vi "DPT Save to Excel.vi"(4 "2015 Raw Data":string[][](array[string]), 6 "Summary":string="*****  2015 DRYER D.O.E. AUDIT DATA WORKSHEET   *****\n\n    Technician:  Corey\t\t\t\tModel #: GSH25J\n    Date:  11/19/1984\t\t\t                Serial #: 96060225101          \t\t\n    Energy Cloth Type:\t  ____________\t\tMfg Date: ____________         \t\n    Blower Type:  _________________\t\tRm. Dry Bulb: F       \n    Blower Dia:  ____________  IN\t\tRm. Wet Bulb:____________F         \n    Airflow (AHAM Sim):  _______CFM\t\tRm. Rel Humidity:   %       \n    Drying Cycle:  ________________\t\tHIGH HEAT_________________________\n    Load Cycles:  \t                (LIMIT 25, WEIGH BONE DRY EVERY 5th RUN)\n    Washer Water Temperature ( 60 ± 5°F ): \n    Exhaust Type: \n    Equipment Calibration: Reference Spreadsheet File\n\n    \tTotal Drying Time:     41.7  min\n(A) \tBone Dry Weight:       8.338 lb\t\t\t(ALL WEIGHTS FROM REF SCALE)\n(B) \tInitial Wt. Wet Load:  13.126  lb\t\t(C) Initial Ret. 100*(B-A)/A:  57.42 %\n(D) \tFinal Wt. Dried Load:  8.686  lb\t\t(E) Final Ret.   100*(D-A)/A:  4.17 %\n\nELECTRICAL ENERGY:\n\n(F) Electrical Energy Used:  0.139  kwh\n\nGAS ENERGY:\n\n\tGas Meter Temp:   73.400 F\t   (H) Gas Corr. Factor:     0.810  ++ \n\tGas Meter Press:  7.700 in H20      (J) Gas Heating Value:    1010.0  BTU/CUFT           \n(G) Metered Gas Vol:      248.500 Liters (K) Gas Energy (G*H*J*0.0353):     7182.0 BTU\t     \n           \nBarometer Press:  24.362 in HG\t           Supply Voltage: \t\n\nReference Pressure: 14.730                    Reference Temperature: 60.0\n\n++ From PC program per US Bureau of Stds, C417,1938\n \n(N) Total Energy (Gas + Electric) (kWh): 2.242\n    [(K/3415)+F]\n\n(L) Per cycle Total Electric Energy Consumption adjusted to 4%:  2.343 KWH/CYCLE\n    ([53.5/(C-E)]*1.04*N)\n\n(I) Per Cycle Off Mode/Standby Mode Power: 0.12\n    [V/(1000*283)*8620] \n\n(V) Standby Mode Power: 3.960 Watts\n    Off Mode Power: 0.000 Watts \n         Off Mode > 0  Standby Mode > 0: [0.5*(Off Mode+Standby Mode)]\n         Off Mode > 0  Standby Mode = 0: [(Off Mode+Standby Mode)]\n\n(E60) Annual Consumption: [(L*283)]  663 kwh\n\n(R) Combined Energy Factor: [A/(L+I)] 3.384\n\n***********************************************************\n   * (P) Per Cycle Energy Efficiency (A/L): 3.559\n***********************************************************", 7 "Pass Fail Lab Eval":string, 8 "error in (no error)":errorcluster, 9 "FileInit Cluster":T1={"Dryer Type"="NR", "TR Number"="", "Lab ID"="", "Output Stream Header"=[], "Stream Data Output"=[], "2015 Array"=[], "Dryer Test Data"=[], "Off Mode Array"=[], "Calibration Array"=[], "File Initialization Array"=[], "Load Run Number"="", "Model:"="DGnn", "Serial Number:"="DGnn", "Build:"="", "Test_Title Per TR:"="HeatUP", "Ambient Temp SetPoint:"="70", "Washer Water \nTemperature ( 60 ± 5°F ):"="60", "Frequency:"="60 HZ", "Dryness Setting:"="", "Heat Setting:"="", "Ambient RH:"="50", "Drying Cycle:"="", "Exhaust:"="NR", "Comments:"="", "Technician:"="", "Engineer:"="CraigT.", "Water Hardness (PPM)"="60", "Empty Dryer Cold Weight"="HeatUP", "Date:"="DGnn", "Version:"="DGnn", "Computer:"="1A", "Load Type"="", "Nominal Load  Weight"="", "Weights Out"={"Measured IMC"=7.0, "Actual RMC"=7.0, "RMC (Desired)"=100.0, "Bone Dry Wt(lbs)"=7.0, "Tolerance(%)"=5.0}, "Test Station:"="1A", "Heat Setting:"="", "Dryness Setting:"="", "Frequency:"="60 HZ", "Water Hardness (PPM)"="60", "Washer Water \nTemperature ( 60 ± 5°F )"="60", "Flow Computer Info Baro,BTUF,u,Z"=[], "Filename"="", "Analog Voltage Data"=[]} {"Weights Out"."Tolerance(%)" format="%0#_6g"; "Weights Out"."Bone Dry Wt(lbs)" format="%03_6g"; "Weights Out"."RMC (Desired)" format="%0#_6g"; "Weights Out"."Actual RMC" format="%03_6g"; "Weights Out"."Measured IMC" format="%0#_6g"}, 10 "report file path":path, 11 "template (empty)":path) -> (0 "error out":errorcluster, 3 "Error":errorcluster[](array[cluster]))   [LabVIEW 2016]
uses:
  Utility/Save File/File Setup (Public)/Type Definition/DPT Output Dryer Information.ctl
  <vilib>/addons/_office/_exclsub.llb/font.ctl
  <vilib>/addons/_office/excel.llb/Excel Easy Table (str).vi
  <vilib>/Utility/NIReport.llb/NI_report.lvclass
  <vilib>/Utility/NIReport.llb/Excel/NI_Excel.lvclass
  <vilib>/addons/_office/NI_ReportGenerationToolkit.lvlib
  Utility/Save File/File Setup.lvlib
panel:
  in  "Machine Debug Information":string[][](array[string])
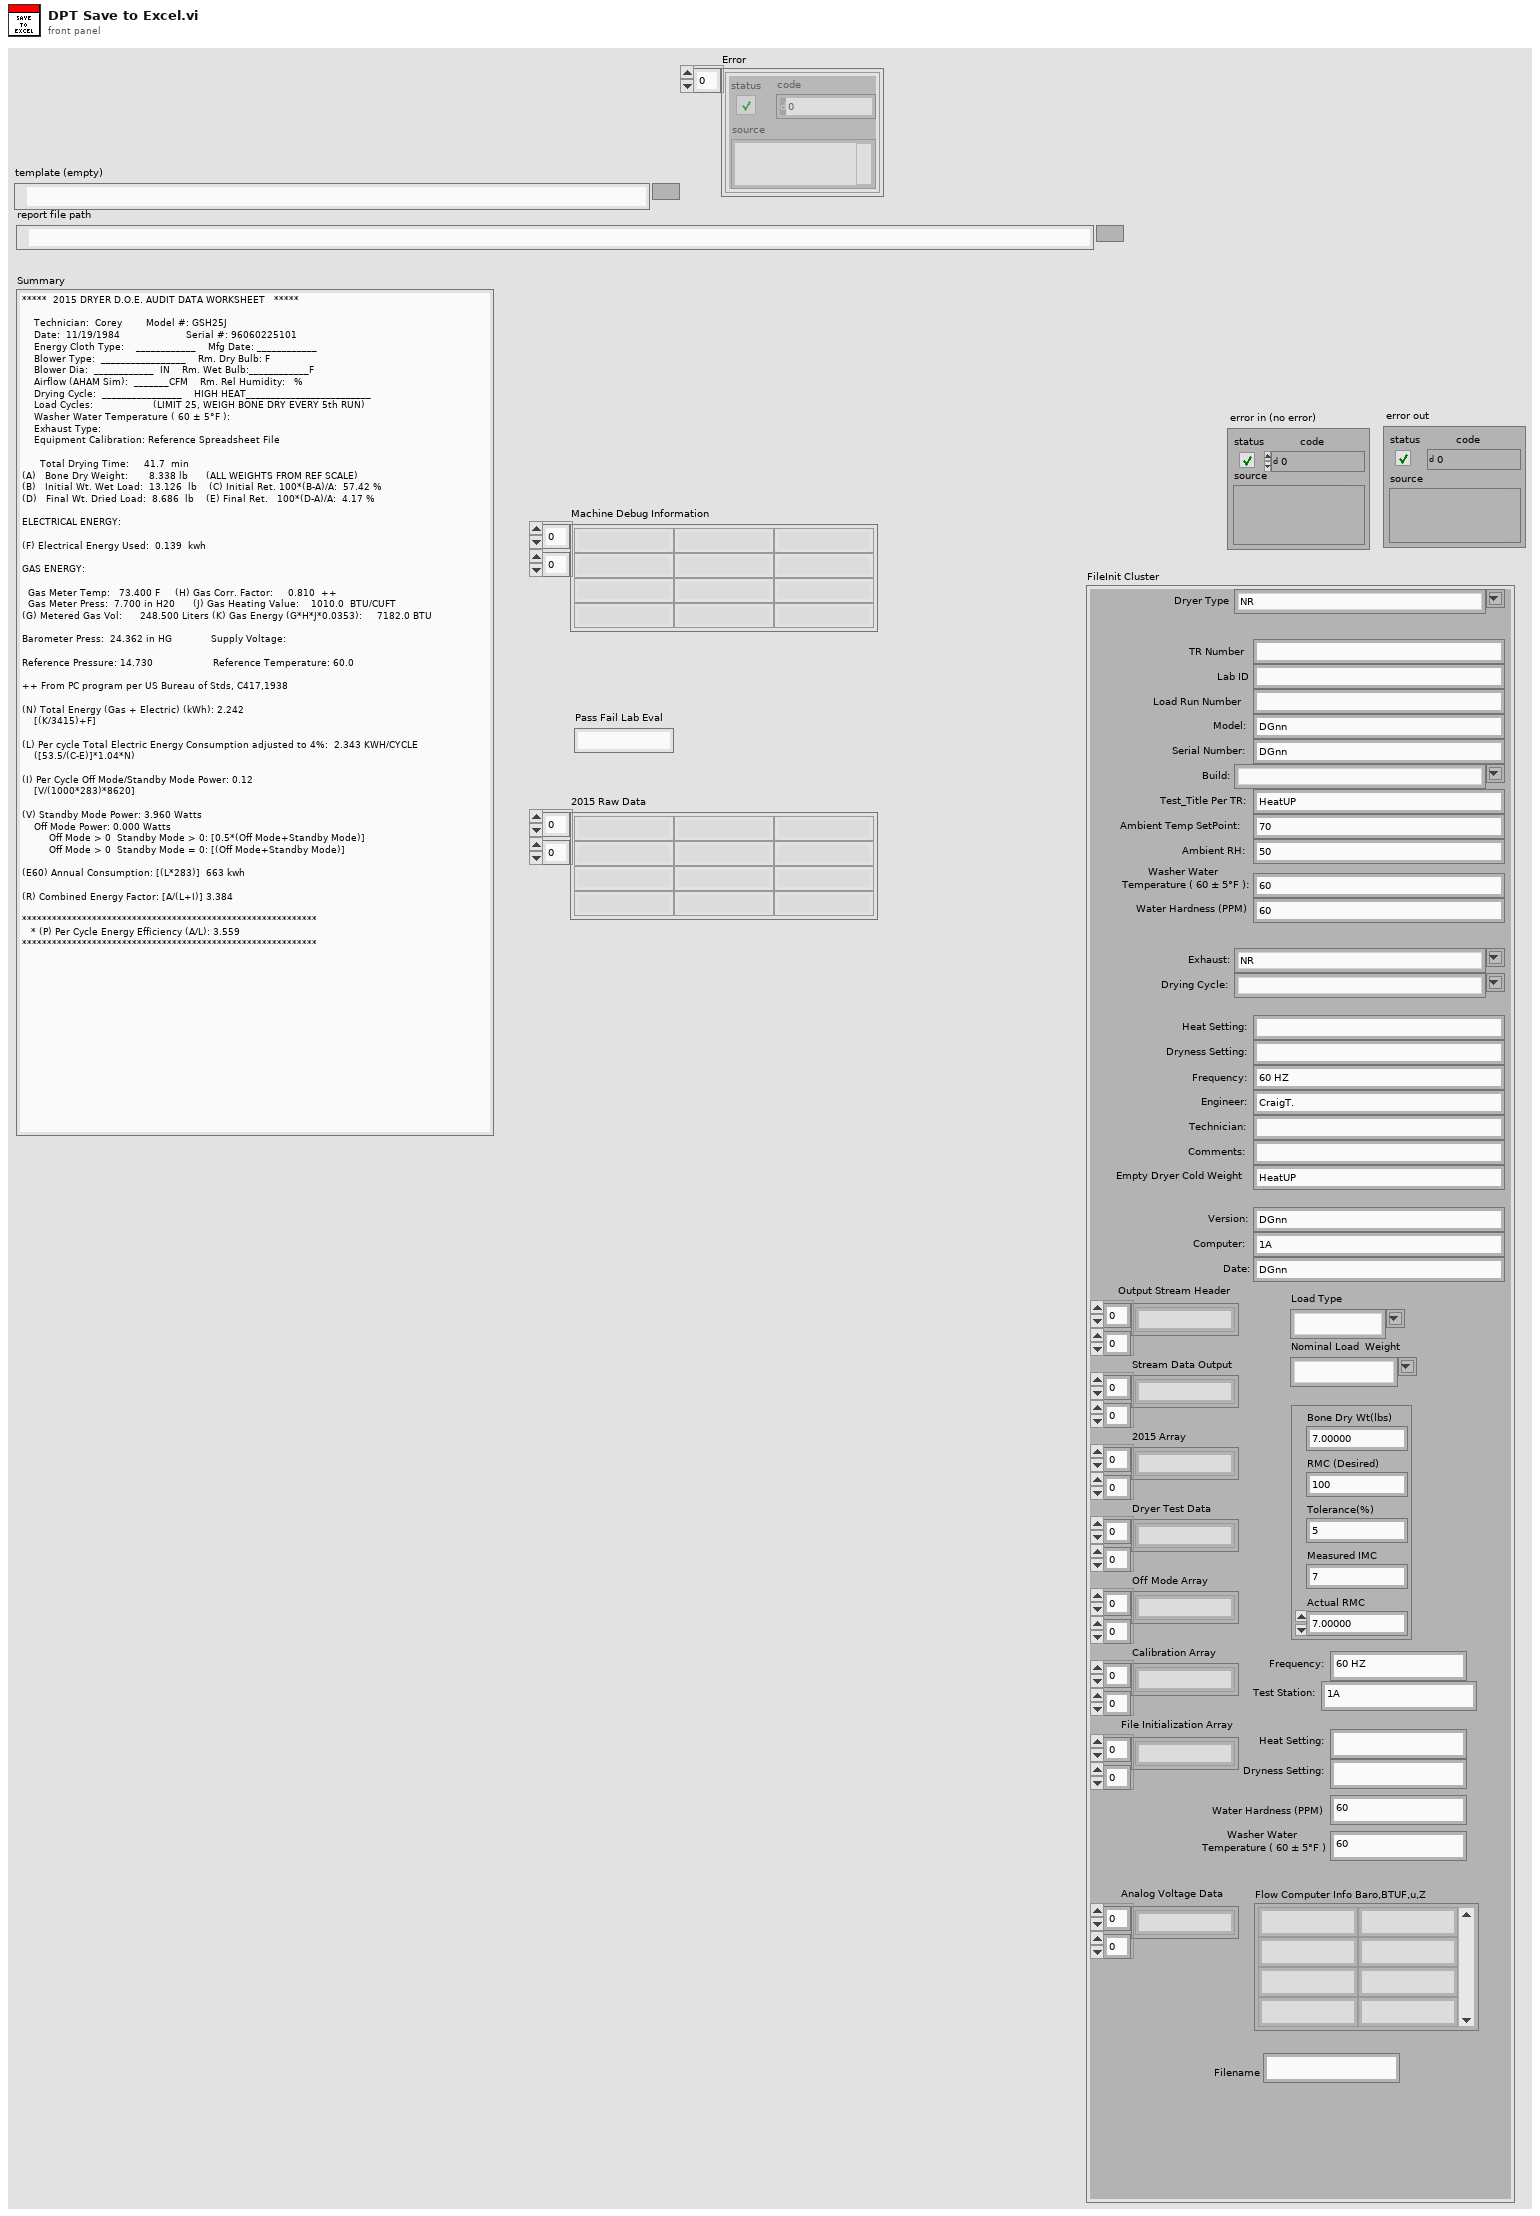
[diagram p1: front panel]
types:
  T1 = typedef "File Setup.lvlib/DPT Output Dryer Information.ctl" = cluster{"Dryer Type":string, "TR Number":string, "Lab ID":string, "Output Stream Header":string[][], "Stream Data Output":string[][], "2015 Array":string[][], "Dryer Test Data":string[][], "Off Mode Array":string[][], "Calibration Array":string[][], "File Initialization Array":string[][], "Load Run Number":string, "Model:":string, "Serial Number:":string, "Build:":string, "Test_Title Per TR:":string, "Ambient Temp SetPoint:":string, "Washer Water \nTemperature ( 60 ± 5°F ):":string, "Frequency:":string, "Dryness Setting:":string, "Heat Setting:":string, "Ambient RH:":string, "Drying Cycle:":string, "Exhaust:":string, "Comments:":string, "Technician:":string, "Engineer:":string, "Water Hardness (PPM)":string, "Empty Dryer Cold Weight":string, "Date:":string, "Version:":string, "Computer:":string, "Load Type":string, "Nominal Load  Weight":string, "Weights Out":cluster{"Measured IMC":dbl, "Actual RMC":dbl, "RMC (Desired)":dbl, "Bone Dry Wt(lbs)":dbl, "Tolerance(%)":dbl}, "Test Station:":string, "Heat Setting:":string, "Dryness Setting:":string, "Frequency:":string, "Water Hardness (PPM)":string, "Washer Water \nTemperature ( 60 ± 5°F )":string, "Flow Computer Info Baro,BTUF,u,Z":string[][], "Filename":string, "Analog Voltage Data":string[][]}
  T2 = typedef "NI_ReportGenerationToolkit.lvlib/font.ctl" = cluster{"font name":string, "font size":dbl, "bold":u16, "italic":u16, "underline":u16, "strike through":u16, "font color":u32}
  T3 = enum16{"maximized", "minimized", "normal", "no change"}
  T4 = enum16{"Standard Report", "HTML", "Word", "Excel"}
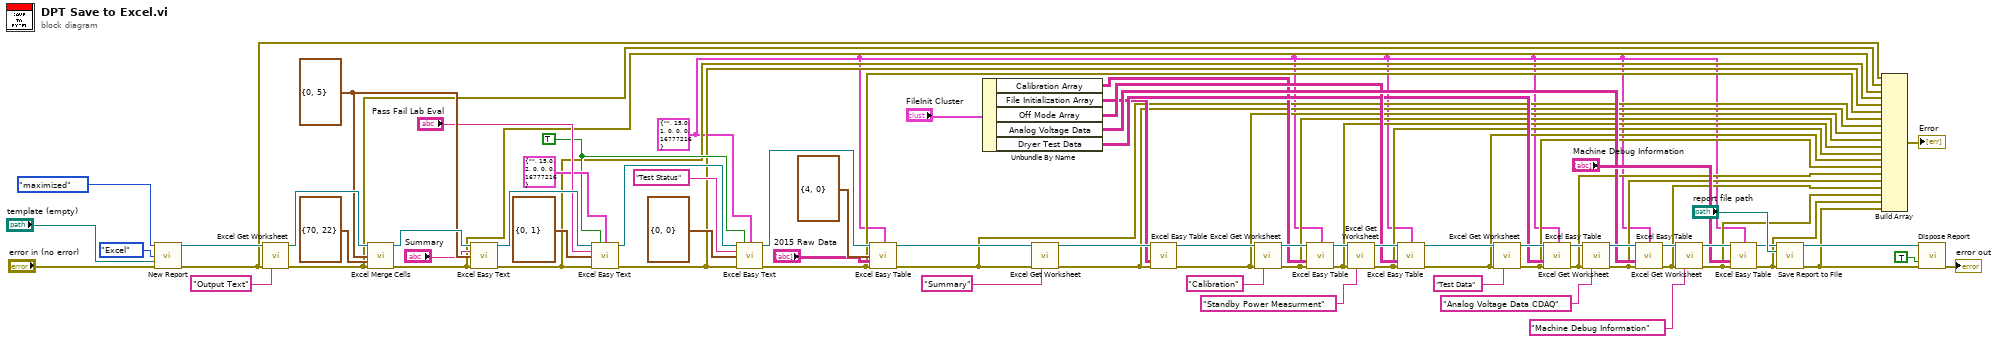
[diagram p0: block diagram]
diagram:
  w1 = T2 {"font name"="", "font size"=15.0, "bold"=1, "italic"=0, "underline"=0, "strike through"=0, "font color"=16777216} ("font")
  w42 = TRUE ("border? (F)")
  w64 = cluster{"row":i32, "column":i32} {"row"=0, "column"=5} ("start (-1, -1)")
  n1 = call <vilib>:"New Report.vi"("window state (normal)"=T3."maximized", "report type"=T4."Excel", "template (empty)"="template (empty)", "error in (no error)"="error in (no error)") -> ("report out"=w68:refnum<class "NI_report.lvclass">, "error out"=w22:errorcluster)  [unwired: 10 in]
  n2 = call <vilib>:"Excel Get Worksheet.vi"("report in"=w68, "error in (no error)"=w22, "name (\"\")"="Output Text" ("name (\"\")")) -> ("report out"=w67:refnum<class "NI_report.lvclass">, "error out"=w21:errorcluster)  [unwired: 11 in]
  n3 = call <vilib>:"Excel Merge Cells.vi"("report in"=w67, "start (-1, -1)"=w64, "end (-1, -1)"=cluster{"row":i32, "column":i32} {"row"=70, "column"=22}, "error in (no error)"=w21) -> ("report out"=w65:refnum<class "NI_report.lvclass">, "error out"=w20:errorcluster)  [unwired: 10 in]
  n4 = call <vilib>:"Excel Easy Text.vi"("report in"=w65, "text"="Summary", "start (-1, -1)"=w64, "error in (no error)"=w20) -> ("report out"=w62:refnum<class "NI_report.lvclass">, "error out"=w19:errorcluster)  [unwired: 7 in, 3 out]
  n5 = call <vilib>:"Excel Easy Text.vi"("report in"=w62, "border? (F)"=w42, "font"=T2 {"font name"="", "font size"=15.0, "bold"=2, "italic"=0, "underline"=0, "strike through"=0, "font color"=16777216}, "text"="Pass Fail Lab Eval", "start (-1, -1)"=cluster{"row":i32, "column":i32} {"row"=0, "column"=1}, "error in (no error)"=w19) -> ("report out"=w43:refnum<class "NI_report.lvclass">, "error out"=w18:errorcluster)  [unwired: 5 in, 3 out]
  n6 = call <vilib>:"Excel Easy Text.vi"("report in"=w43, "border? (F)"=w42, "font"=w1, "text"="Test Status", "start (-1, -1)"=cluster{"row":i32, "column":i32} {"row"=0, "column"=0}, "error in (no error)"=w18) -> ("report out"=w26:refnum<class "NI_report.lvclass">, "error out"=w17:errorcluster)  [unwired: 5 in, 3 out]
  n7 = call-poly <vilib>:"Excel Easy Table.vi"("report in"=w26, "font"=w1, "start (0, 0)"=cluster{"row":i32, "column":i32} {"row"=4, "column"=0}, "text data"="2015 Raw Data", "error in (no error)"=w17) -> ("report out"=w25:refnum<class "NI_report.lvclass">, "error out"=w16:errorcluster)  [unwired: 6 in, 3 out]
  n8 = Unbundle By Name("FileInit Cluster") -> ("Calibration Array"=w30:string[][], "File Initialization Array"=w34:string[][], "Off Mode Array"=w38:string[][], "Analog Voltage Data"=w39:string[][], "Dryer Test Data"=w37:string[][])
  n9 = call <vilib>:"Excel Get Worksheet.vi"("report in"=w25, "error in (no error)"=w16, "name (\"\")"="Summary" ("name (\"\")")) -> ("report out"=w35:refnum<class "NI_report.lvclass">, "error out"=w15:errorcluster)  [unwired: 11 in]
  n10 = call-poly <vilib>:"Excel Easy Table.vi"("report in"=w35, "text data"=w34, "error in (no error)"=w15) -> ("report out"=w33:refnum<class "NI_report.lvclass">, "error out"=w14:errorcluster)  [unwired: 8 in, 3 out]
  n11 = call <vilib>:"Excel Get Worksheet.vi"("report in"=w33, "error in (no error)"=w14, "name (\"\")"="Calibration" ("name (\"\")")) -> ("report out"=w31:refnum<class "NI_report.lvclass">, "error out"=w13:errorcluster)  [unwired: 11 in]
  n12 = call-poly <vilib>:"Excel Easy Table.vi"("report in"=w31, "font"=w1, "text data"=w30, "error in (no error)"=w13) -> ("report out"=w29:refnum<class "NI_report.lvclass">, "error out"=w12:errorcluster)  [unwired: 7 in, 3 out]
  n13 = call <vilib>:"Excel Get Worksheet.vi"("report in"=w29, "error in (no error)"=w12, "name (\"\")"="Standby Power Measurment" ("name (\"\")")) -> ("report out"=w59:refnum<class "NI_report.lvclass">, "error out"=w11:errorcluster)  [unwired: 11 in]
  n14 = call-poly <vilib>:"Excel Easy Table.vi"("report in"=w59, "font"=w1, "text data"=w38, "error in (no error)"=w11) -> ("report out"=w47:refnum<class "NI_report.lvclass">, "error out"=w10:errorcluster)  [unwired: 7 in, 3 out]
  n15 = call <vilib>:"Excel Get Worksheet.vi"("report in"=w47, "error in (no error)"=w10, "name (\"\")"="Test Data" ("name (\"\")")) -> ("report out"=w56:refnum<class "NI_report.lvclass">, "error out"=w9:errorcluster)  [unwired: 11 in]
  n16 = call-poly <vilib>:"Excel Easy Table.vi"("report in"=w56, "font"=w1, "text data"=w37, "error in (no error)"=w9) -> ("report out"=w55:refnum<class "NI_report.lvclass">, "error out"=w8:errorcluster)  [unwired: 7 in, 3 out]
  n17 = call <vilib>:"Excel Get Worksheet.vi"("report in"=w55, "error in (no error)"=w8, "name (\"\")"="Analog Voltage Data CDAQ" ("name (\"\")")) -> ("report out"=w53:refnum<class "NI_report.lvclass">, "error out"=w7:errorcluster)  [unwired: 11 in]
  n18 = call-poly <vilib>:"Excel Easy Table.vi"("report in"=w53, "font"=w1, "text data"=w39, "error in (no error)"=w7) -> ("report out"=w52:refnum<class "NI_report.lvclass">, "error out"=w6:errorcluster)  [unwired: 7 in, 3 out]
  n19 = call <vilib>:"Excel Get Worksheet.vi"("report in"=w52, "error in (no error)"=w6, "name (\"\")"="Machine Debug Information" ("name (\"\")")) -> ("report out"=w50:refnum<class "NI_report.lvclass">, "error out"=w5:errorcluster)  [unwired: 11 in]
  n20 = call-poly <vilib>:"Excel Easy Table.vi"("report in"=w50, "font"=w1, "text data"="Machine Debug Information", "error in (no error)"=w5) -> ("report out"=w48:refnum<class "NI_report.lvclass">, "error out"=w4:errorcluster)  [unwired: 7 in, 3 out]
  n21 = call-dynamic "Save Report to File.vi"("report in"=w48, "report file path"="report file path", "error in (no error)"=w4) -> ("report out"=w71:refnum<class "NI_report.lvclass">, "error out"=w3:errorcluster)  [unwired: 11 in]
  n22 = Build Array(w22, w21, w20, w19, w18, w17, w16, w15, w14, w13, w12, w11, w10, w9, w8, w7, w6, w5, w4, w3) -> (→"Error":errorcluster[])
  n23 = call-dynamic "Dispose Report.vi"("report in"=w71, "save changes? (F)"=TRUE, "error in (no error)"=w3) -> ("error out"=→"error out":errorcluster)  [unwired: 12 in]
